vi "Spreadsheet1.vi"   [LabVIEW 2020]
uses:
  <vilib>/Utility/NIReport.llb/Report Type.ctl
  <vilib>/addons/_office/excel.llb/Excel Easy Table (str).vi
  <vilib>/Utility/NIReport.llb/NI_report.lvclass
  <vilib>/addons/_office/NI_ReportGenerationToolkit.lvlib
  <vilib>/Utility/NIReport.llb/NI_ReportGenerationCore.lvlib
types:
  T1 = typedef "NI_ReportGenerationCore.lvlib/Report Type.ctl" = enum16{"HTML", "Word", "Excel"}
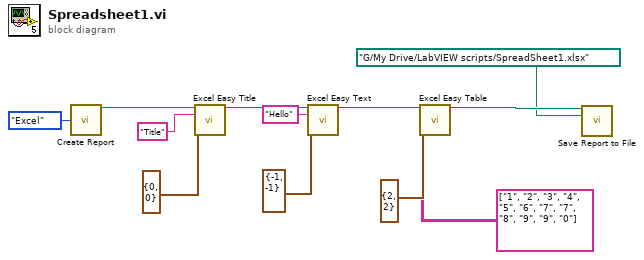
[diagram p0: block diagram]
diagram:
  n1 = call <vilib>:"Create Report.vi"("report type"=Report_Type."Excel") -> ("report out"=w12:refnum<class "NI_report.lvclass">)  [unwired: 13 in, 1 out]
  n2 = call <vilib>:"Excel Easy Title.vi"("report in"=w12, "title"="Title", "start (0, 0)"=cluster{"row":i32, "column":i32} {"row"=0, "column"=0}) -> ("report out"=w11:refnum<class "NI_report.lvclass">)  [unwired: 10 in, 2 out]
  n3 = call <vilib>:"Excel Easy Text.vi"("report in"=w11, "text"="Hello", "start (-1, -1)"=cluster{"row":i32, "column":i32} {"row"=-1, "column"=-1}) -> ("report out"=w10:refnum<class "NI_report.lvclass">)  [unwired: 8 in, 4 out]
  n4 = call-poly <vilib>:"Excel Easy Table.vi"("report in"=w10, "start (0, 0)"=cluster{"row":i32, "column":i32} {"row"=2, "column"=2}, "text data"=string[][] [["1", "2", "3", "4"], ["5", "6", "7", "7"], ["8", "9", "9", "0"]]) -> ("report out"=w9:refnum<class "NI_report.lvclass">)  [unwired: 8 in, 4 out]
  n5 = call-dynamic "Save Report to File.vi"("report in"=w9, "report file path"=path "G:/My Drive/LabVIEW scripts/SpreadSheet1.xlsx") -> ()  [unwired: 12 in, 2 out]
